vi "Navigation_Main_r1.vi"() -> ()   [LabVIEW 2015]
uses:
  <vilib>/myRIO/Instrument Drivers/Onboard IO/PWM/typedefs/PWM Reference.ctl
  <vilib>/myRIO/Common/Instrument Driver Framework/Utilities/typedefs/myRIO Generic Hardware Reference.ctl
  <vilib>/myRIO/Common/Instrument Driver Framework/Utilities/typedefs/Hardware Version Enum.ctl
  <vilib>/myRIO/Common/Instrument Driver Framework/Utilities/typedefs/myRIO v1.0 Reference.ctl
  <vilib>/myRIO/Common/Instrument Driver Framework/Utilities/typedefs/Generic FPGA Reference.ctl
  <vilib>/myRIO/Common/Instrument Driver Framework/myRIO v1.0/PWM/typedefs/PWM Channels Enum.ctl
  <vilib>/myRIO/Instrument Drivers/Onboard IO/PWM/typedefs/PWM Configuration.ctl
  <vilib>/userdefined/High Color/nirio_resource_hc.ctl
  <vilib>/myRIO/Common/Instrument Driver Framework/myRIO v1.0/PWM/vis/myRIO v1.1 Open PWM.vi
  <vilib>/myRIO/Common/Instrument Driver Framework/Utilities/vis/Validate Channels.vi
  <vilib>/myRIO/Common/Instrument Driver Framework/myRIO v1.0/PWM/vis/myRIO v1.0 Reserve PWM.vi
  <vilib>/myRIO/Common/Instrument Driver Framework/myRIO v1.0/PWM/vis/myRIO v1.0 Close PWM.vi
  <vilib>/myRIO/Common/Instrument Driver Framework/myRIO v1.0/PWM/vis/myRIO v1.0 Build MUX Configuration PWM.vi
  <vilib>/myRIO/Common/Instrument Driver Framework/myRIO v1.0/Resource Manager/vis/myRIO v1.0 Reserve Channel List.vi
  <vilib>/myRIO/Common/Instrument Driver Framework/myRIO v1.0/PWM/vis/myRIO v1.0 Unreserve PWM.vi
  <vilib>/myRIO/Common/Instrument Driver Framework/myRIO v1.0/Resource Manager/vis/myRIO v1.0 Create Configuration List.vi
  <vilib>/myRIO/Common/Instrument Driver Framework/myRIO v1.0/Resource Manager/vis/myRIO v1.0 Reserve Channel.vi
  <vilib>/myRIO/Common/Instrument Driver Framework/myRIO v1.0/Resource Manager/vis/myRIO v1.0 Unreserve Channel.vi
  <vilib>/myRIO/Common/Instrument Driver Framework/myRIO v1.0/Resource Manager/vis/myRIO v1.0 Unreserve Channel List.vi
  <vilib>/myRIO/Common/Instrument Driver Framework/myRIO v1.0/Resource Manager/vis/myRIO v1.0 Build Mutex Name.vi
  <vilib>/FPGAPlugInAG/myRIO-1900/niLvFpga_Open_myRIO-1900.vi
  <vilib>/rvi/interface/common/dynamic/niFpgaDynamicAddResources.vi
  <vilib>/myRIO/Common/Instrument Driver Framework/Utilities/vis/FPGA Ref Manager.vi
  <vilib>/Utility/error.llb/Error Cluster From Error Code.vi
  <vilib>/myRIO/Common/Instrument Driver Framework/Utilities/vis/Ref Counter.vi
  <vilib>/rvi/errors/niLvFpgaAdjustHostInterfaceError.vi
  <vilib>/Utility/VariantDataType/GetNumericInfo.vi
  <vilib>/myRIO/Common/Instrument Driver Framework/myRIO v1.0/myRIO v1.1 Open.vi
  <vilib>/myRIO/Common/Instrument Driver Framework/Utilities/vis/IO Manager.vi
  <vilib>/myRIO/Common/Instrument Driver Framework/Utilities/vis/Configuration Manager.vi
  <vilib>/myRIO/Common/Instrument Driver Framework/myRIO v1.0/Resource Manager/vis/myRIO v1.0 Configure IO.vi
  <vilib>/myRIO/Common/Instrument Driver Framework/myRIO v1.0/myRIO v1.0 Close.vi
  <vilib>/myRIO/Common/Instrument Driver Framework/myRIO v1.0/PWM/vis/myRIO v1.0 Write PWM.vi
  <vilib>/myRIO/Common/Instrument Driver Framework/myRIO v1.0/PWM/vis/myRIO v1.0 Shutdown PWM.vi
  <vilib>/rvi/interface/nirviOpenFPGA/nirviOpenFPGA.xnode
  Navi/E/FPGA Bitfiles/NavigationProjec_FPGATarget2_FPGAMainNavigati_PWPHW8gwDxI.lvbitx
  <vilib>/rvi/interface/nirviReadWriteControl/nirviReadWriteControl.xnode
  <vilib>/myRIO/Instrument Drivers/Onboard IO/PWM/vis/myRIO PWM Open.xnode
  <vilib>/myRIO/Instrument Drivers/Onboard IO/PWM/PWM.lvlib
  <vilib>/myRIO/Instrument Drivers/Utilities/Utilities.lvlib
  NiFpgaLv.dll
  <vilib>/rvi/interface/Simulation/niFpgaSimulationCallBeginRW.vi
panel:
  out "tan(x)":dbl
  in  "x":dbl
  out "X Distance Taveled":dbl
  out "Y Distance Traveled":dbl
  out "Left ENC Avg":dbl
  out "Right ENC Avg":dbl
  out "Distance Traveled":dbl
  out "X Current Position":dbl
  out "Y Current Position":dbl
  out "Reset X Y":dbl
  out "Tick Count(mSec) 2":u32 caption="Tick Count(mSec)"
  out "Right Setpoint":dbl
  out "Left Setpoint":dbl
  out "Scale":dbl=1.0
  in  "Go":bool
  in  "Start Position Y":dbl=5.0
  in  "Goal Position X":dbl=20.0
  in  "Start Position X":dbl=1.0
  in  "All Stop":bool
  in  "Left Side PID Gains":T1={"proportional gain (Kc)"=0.002, "integral time (Ti, min)"=7e-07, "derivative time (Td, min)"=0.0} {"derivative time (Td, min)" format="%.8f"; "integral time (Ti, min)" format="%.8f"; "proportional gain (Kc)" format="%.8f"}
  in  "Left Side Output Range":cluster{"output high":dbl, "output low":dbl}={"output high"=0.13333, "output low"=-0.13333} {"output low" format="%.5f"; "output high" format="%.5f"}
  in  "Right Side PID Gains":T1={"proportional gain (Kc)"=0.002, "integral time (Ti, min)"=7e-07, "derivative time (Td, min)"=0.0} {"derivative time (Td, min)" format="%.8f"; "integral time (Ti, min)" format="%.8f"; "proportional gain (Kc)" format="%.8f"}
  in  "Right Side Output Range":cluster{"output high":dbl, "output low":dbl}={"output high"=0.13333, "output low"=-0.13333} {"output low" format="%.5f"; "output high" format="%.5f"}
  out "Left PWM":dbl
  out "Right PWM":dbl
  out "LF Rot Velocity (rot/s)":dbl
  out "LM Rot Velocity (rot/s)":dbl
  out "LR Rot Velocity (rot/s)":dbl
  out "RR Rot Velocity (rot/s)":dbl
  out "RM Linear Velocity (rot/s)":dbl
  out "RF Linear Velocity (rot/s)":dbl
  in  "Encoder Reset":bool
  out "SYS.SELECTA":u8 format="%08b"
  out "ENC.B_c.CNTR":i32
  out "ENC.B_b.CNTR":i32
  out "ENC.B_a.CNTR":i32
  out "ENC.A_c.CNTR":i32
  out "ENC.A_b.CNTR":i32
  out "ENC.A_a.CNTR":i32
  out "Current Rot Velocity (rot/s)":T2(graph)
  # "Motor Control Parameters"
  # "Press Go when Start and Goal Are Set"
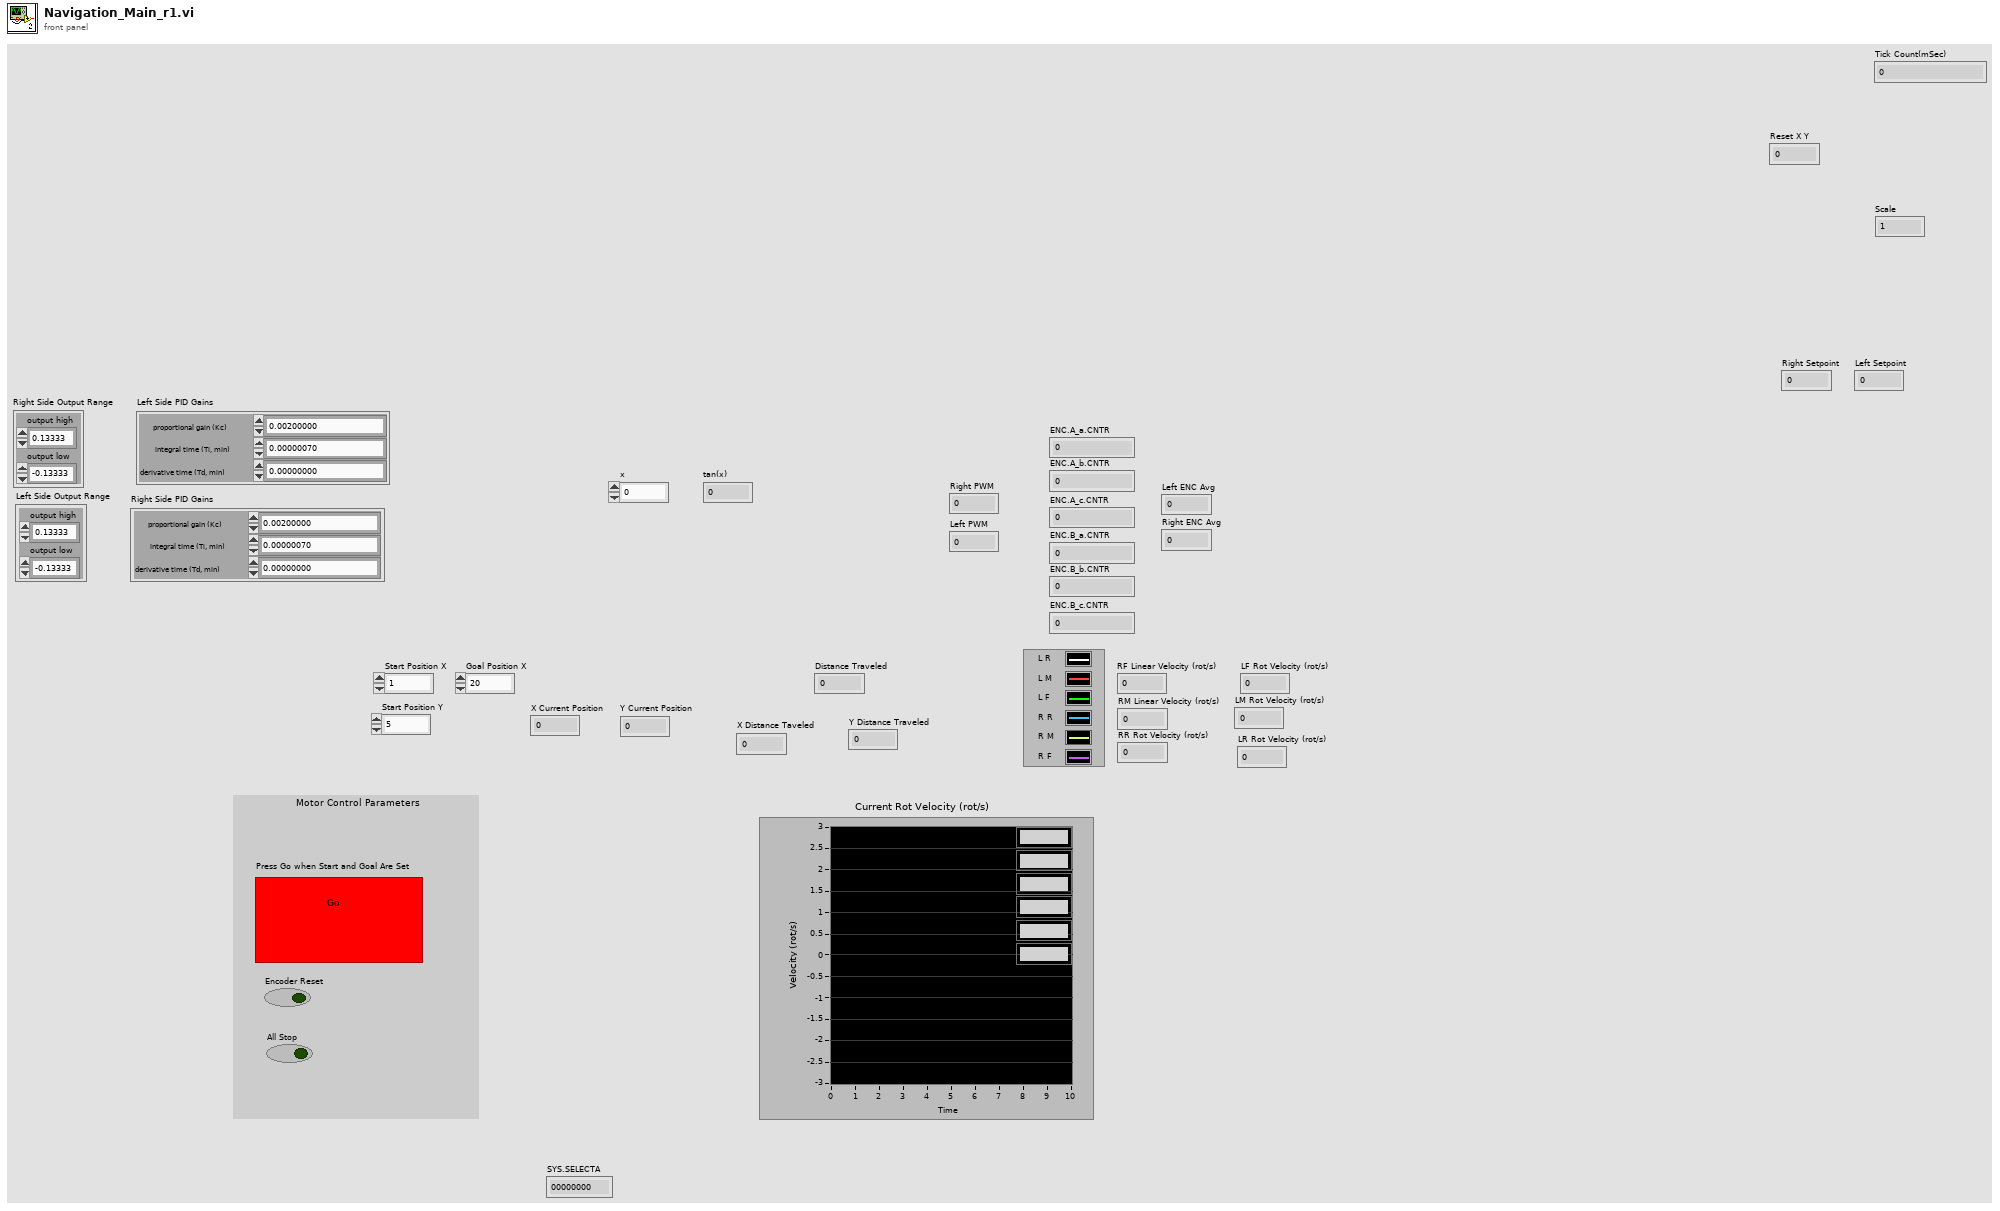
[diagram p1: front panel]
types:
  T1 = cluster{"proportional gain (Kc)":dbl, "integral time (Ti, min)":dbl, "derivative time (Td, min)":dbl}
  T2 = cluster{"Rotational Velocity (RPS)":dbl, "Rotational Velocity (RPS)":dbl, "Rotational Velocity (RPS)":dbl, "Rotational Velocity (RPS)":dbl, "Rotational Velocity (RPS)":dbl, "Rotational Velocity (RPS)":dbl}
  T3 = typedef "nirio_resource_hc.ctl" = tag
  T4 = typedef "Hardware Version Enum.ctl" = enum16{"Unknown", "myRIO-1900", "myRIO-1950", "roboRIO"}
  T5 = typedef "PWM.lvlib/PWM Reference.ctl" = cluster{"myRIO Reference":T6, "PWM Channels Enum":T9, "PWM Configuration":T10}
  T6 = typedef "myRIO Generic Hardware Reference.ctl" = cluster{"myRIO Model":T4, "myRIO Hardware Reference":T7}
  T7 = typedef "myRIO v1.0 Reference.ctl" = cluster{"Generic FPGA Reference":T8, "Allow multiple opens":bool}
  T8 = typedef "Generic FPGA Reference.ctl" = refnum<k20>
  T9 = typedef "PWM Channels Enum.ctl" = enum16{"Not Connected", "C/PWM0", "C/PWM1", "A/PWM0", "A/PWM1", "A/PWM2", "B/PWM0", "B/PWM1", "B/PWM2", "PWM/PWM0", "PWM/PWM1", "PWM/PWM2", "PWM/PWM3", "PWM/PWM4", "PWM/PWM5", "PWM/PWM6", "PWM/PWM7", "PWM/PWM8", "PWM/PWM9"}
  T10 = typedef "PWM.lvlib/PWM Configuration.ctl" = cluster{"Frequency":dbl, "Duty Cycle":dbl}
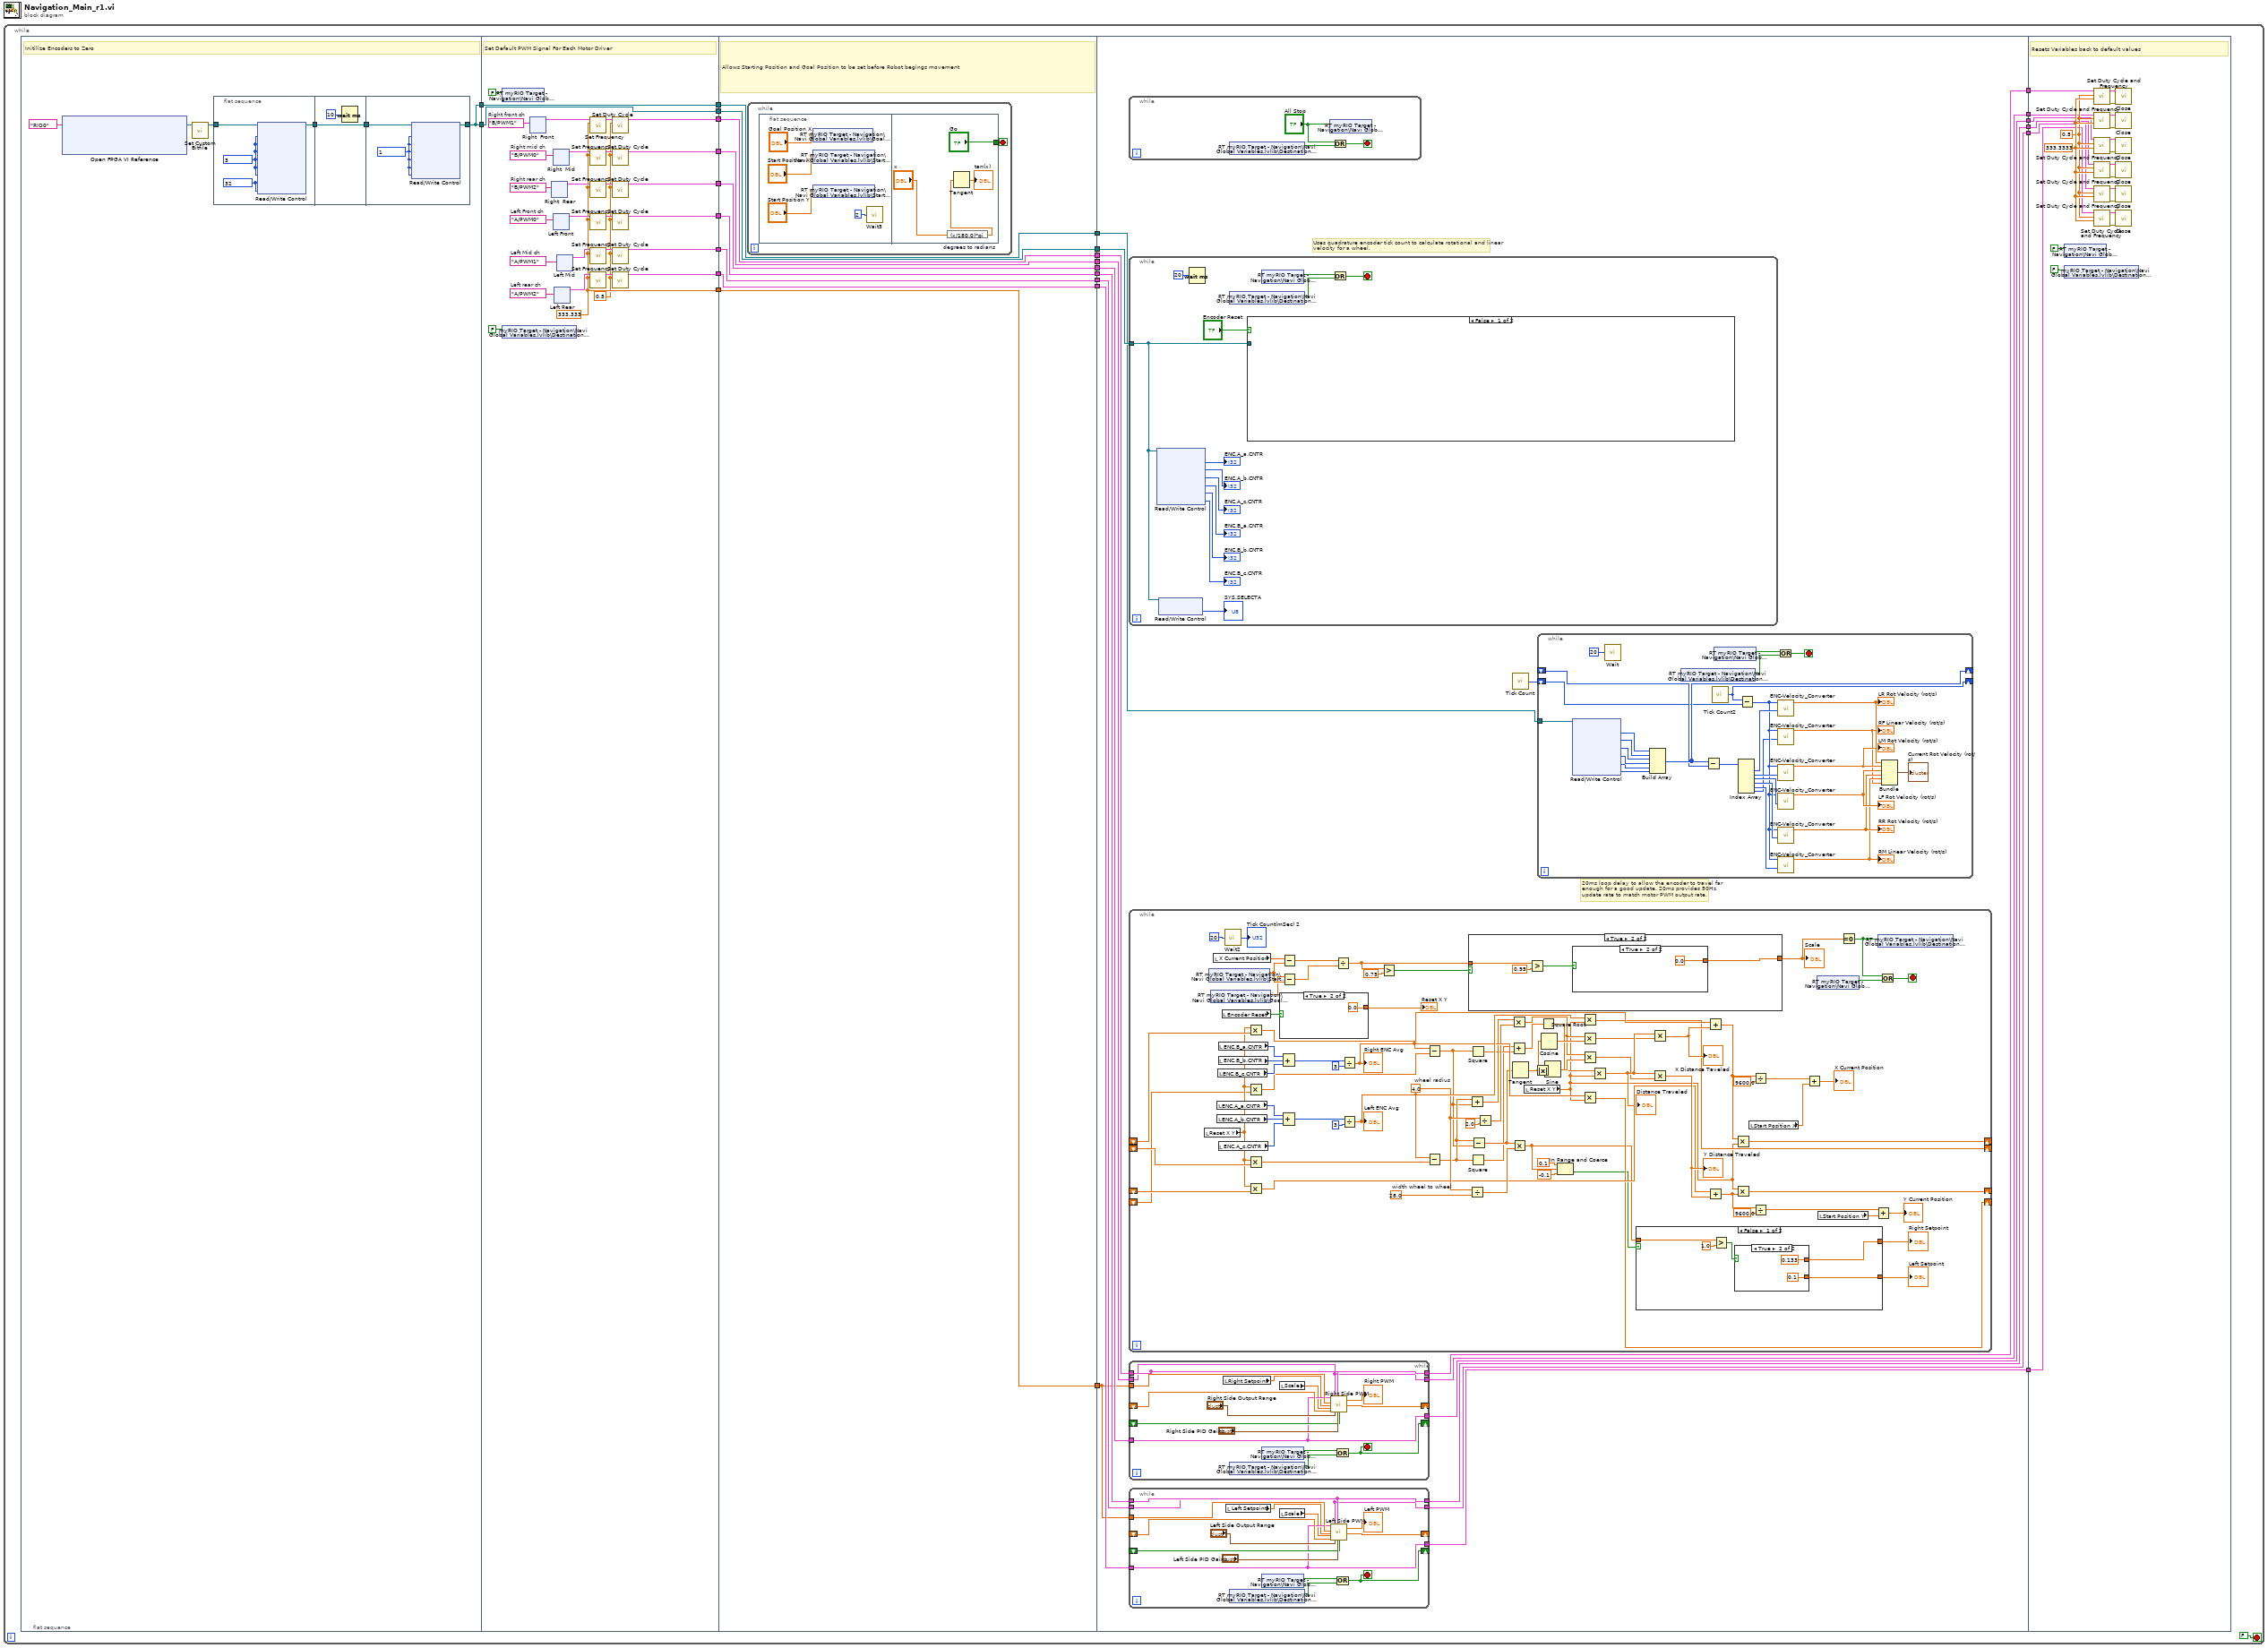
[diagram p0: block diagram]
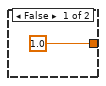
[diagram p2: hidden frame]
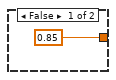
[diagram p3: hidden frame]
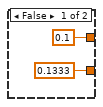
[diagram p4: hidden frame]
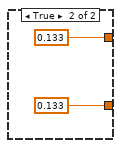
[diagram p5: hidden frame]
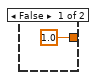
[diagram p6: hidden frame]
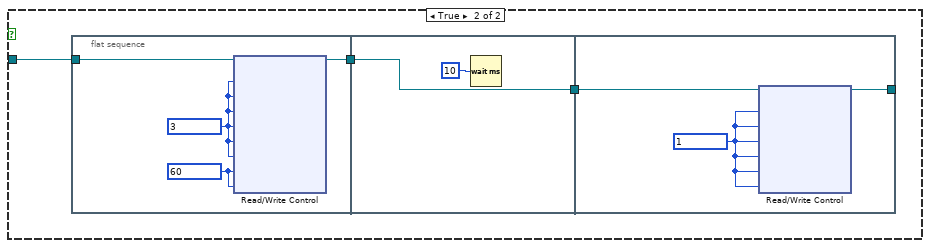
[diagram p7: hidden frame]
diagram:
  n1 = while {
    stop <- FALSE ("stop") stop-if-true
    n2 = flat-sequence {
      tunnel: [w30] -> w27
      tunnel: [w30] -> w26
      tunnel: [w60] -> w25
      tunnel: [w55] -> w24
      tunnel: [w51] -> w23
      tunnel: [w50] -> w22
      tunnel: [w49] -> w21
      tunnel: [w48] -> w20
      tunnel: [w47] -> w19
      tunnel: [w46] -> w18
      tunnel: w27 -> [w45]
      tunnel: [w45] -> w17
      tunnel: w26 -> [w46]
      tunnel: w25 -> [w177]
      tunnel: [w177] -> w16
      tunnel: w24 -> [w176]
      tunnel: [w176] -> w15
      tunnel: w23 -> [w175]
      tunnel: [w175] -> w14
      tunnel: w22 -> [w174]
      tunnel: [w174] -> w13
      tunnel: w21 -> [w173]
      tunnel: [w173] -> w12
      tunnel: w20 -> [w172]
      tunnel: [w172] -> w11
      tunnel: w19 -> [w171]
      tunnel: [w171] -> w10
      tunnel: w18 -> [w170]
      tunnel: [w170] -> w9
      tunnel: w17 -> [w169]
      tunnel: [w169] -> w8
      tunnel: w16 -> [w193]
      tunnel: w15 -> [w194]
      tunnel: w14 -> [w199]
      tunnel: w13 -> [w198]
      tunnel: w12 -> [w197]
      tunnel: w11 -> [w196]
      tunnel: w10 -> [w195]
      tunnel: w9 -> [w201]
      tunnel: w8 -> [w200]
      tunnel: [w192] -> w7
      tunnel: [w191] -> w6
      tunnel: [w190] -> w5
      tunnel: [w189] -> w4
      tunnel: [w188] -> w3
      tunnel: [w187] -> w2
      tunnel: w7 -> [w399]
      tunnel: w6 -> [w398]
      tunnel: w5 -> [w397]
      tunnel: w4 -> [w396]
      tunnel: w3 -> [w395]
      tunnel: w2 -> [w394]
      frame #0 {
        # "Initilize Encoders to Zero"
        n3 = xnode "Open FPGA VI Reference"("resource name"=tag "RIO0") -> ("FPGA VI Reference Out"=w29:refnum<k20>)  [unwired: 1 in, 1 out]
        n4 = call <vilib>:"Set Custom Bitfile.vi"("Custom FPGA Reference In"=w29) -> ("Custom FPGA Reference Out"=w31:refnum<k20>)  [unwired: 9 in, 1 out]
        n5 = flat-sequence {
          tunnel: w31 -> [w36]
          tunnel: [w34] -> w33
          tunnel: w33 -> [w38]
          tunnel: [w38] -> w32
          tunnel: w32 -> [w41]
          tunnel: [w40] -> w30
          frame #0 {
            w35 = u8 32 ("SYS.SELECTA")
            w37 = u8 3 ("ENC.B_c.CNFG")
            n6 = xnode "Read/Write Control"("FPGA VI Reference In"=w36, "ENC.A_a.CNFG"=w37, "ENC.A_b.CNFG"=w37, "ENC.A_c.CNFG"=w37, "ENC.B_a.CNFG"=w37, "ENC.B_b.CNFG"=w37, "ENC.B_c.CNFG"=w37, "SYS.SELECTA"=w35, "SYS.SELECTB"=w35) -> ("FPGA VI Reference Out"=w34:refnum<k20>)  [unwired: 1 in, 1 out]
          }
          frame #1 {
            n7 = Wait (ms)(milliseconds to wait=u32 10) -> ()  [unwired: 1 out]
          }
          frame #2 {
            w42 = u8 1 ("ENC.B_c.CNFG")
            n8 = xnode "Read/Write Control"("FPGA VI Reference In"=w41, "ENC.A_a.CNFG"=w42, "ENC.A_b.CNFG"=w42, "ENC.A_c.CNFG"=w42, "ENC.B_a.CNFG"=w42, "ENC.B_b.CNFG"=w42, "ENC.B_c.CNFG"=w42) -> ("FPGA VI Reference Out"=w40:refnum<k20>)  [unwired: 1 in, 1 out]
          }
        }
      }
      frame #1 {
        w52 = 0.5 ("Duty Cycle")
        w60 = 333.333 ("Frequency [Hz]")
        w67 = tag "B/PWM2"  # Right rear ch
        w68 = tag "B/PWM0"  # Right mid ch
        w69 = tag "B/PWM1"  # Right front ch
        w70 = tag "A/PWM2"  # Left rear ch
        w71 = tag "A/PWM0"  # Left Front ch
        w72 = tag "A/PWM1"  # Left Mid ch
        # "Set Default PWM Signal For Each Motor Driver"
        n9 = shared-variable "RT myRIO Target - Navigation\\Navi Global Variables.lvlib\\All Stop"(FALSE) -> ()  [unwired: 1 in, 1 out]
        n10 = shared-variable "RT myRIO Target - Navigation\\Navi Global Variables.lvlib\\Destination Reached"(FALSE) -> ()  [unwired: 1 in, 1 out]
        n11 = xnode "Right  Front"("Channel Name"=w69) -> ("PWM Ref Out"=w63:T5)  [unwired: 2 in, 1 out]
        n12 = xnode "Right  Rear"("Channel Name"=w67) -> ("PWM Ref Out"=w61:T5)  [unwired: 2 in, 1 out]
        n13 = xnode "Right  Mid"("Channel Name"=w68) -> ("PWM Ref Out"=w62:T5)  [unwired: 2 in, 1 out]
        n14 = xnode "Left Front"("Channel Name"=w71) -> ("PWM Ref Out"=w65:T5)  [unwired: 2 in, 1 out]
        n15 = xnode "Left Rear"("Channel Name"=w70) -> ("PWM Ref Out"=w64:T5)  [unwired: 2 in, 1 out]
        n16 = xnode "Left Mid"("Channel Name"=w72) -> ("PWM Ref Out"=w66:T5)  [unwired: 2 in, 1 out]
        n17 = call <vilib>:"Set Frequency.vi"("Frequency [Hz]"=w60, "PWM Ref In"=w63) -> ("PWM Ref Out"=w56:T5)  [unwired: 7 in, 1 out]
        n18 = call <vilib>:"Set Frequency.vi"("Frequency [Hz]"=w60, "PWM Ref In"=w62) -> ("PWM Ref Out"=w57:T5)  [unwired: 7 in, 1 out]
        n19 = call <vilib>:"Set Frequency.vi"("Frequency [Hz]"=w60, "PWM Ref In"=w61) -> ("PWM Ref Out"=w58:T5)  [unwired: 7 in, 1 out]
        n20 = call <vilib>:"Set Frequency.vi"("Frequency [Hz]"=w60, "PWM Ref In"=w65) -> ("PWM Ref Out"=w53:T5)  [unwired: 7 in, 1 out]
        n21 = call <vilib>:"Set Frequency.vi"("Frequency [Hz]"=w60, "PWM Ref In"=w66) -> ("PWM Ref Out"=w59:T5)  [unwired: 7 in, 1 out]
        n22 = call <vilib>:"Set Frequency.vi"("Frequency [Hz]"=w60, "PWM Ref In"=w64) -> ("PWM Ref Out"=w54:T5)  [unwired: 7 in, 1 out]
        n23 = call <vilib>:"Set Duty Cycle.vi"("Duty Cycle"=w52, "PWM Ref In"=w56) -> ("PWM Ref Out"=w51:T5)  [unwired: 7 in, 1 out]
        n24 = call <vilib>:"Set Duty Cycle.vi"("Duty Cycle"=w52, "PWM Ref In"=w57) -> ("PWM Ref Out"=w50:T5)  [unwired: 7 in, 1 out]
        n25 = call <vilib>:"Set Duty Cycle.vi"("Duty Cycle"=w52, "PWM Ref In"=w58) -> ("PWM Ref Out"=w49:T5)  [unwired: 7 in, 1 out]
        n26 = call <vilib>:"Set Duty Cycle.vi"("Duty Cycle"=w52, "PWM Ref In"=w53) -> ("PWM Ref Out"=w48:T5)  [unwired: 7 in, 1 out]
        n27 = call <vilib>:"Set Duty Cycle.vi"("Duty Cycle"=w52, "PWM Ref In"=w59) -> ("PWM Ref Out"=w47:T5)  [unwired: 7 in, 1 out]
        n28 = call <vilib>:"Set Duty Cycle.vi"("Duty Cycle"=w52, "PWM Ref In"=w54) -> ("PWM Ref Out"=w55:T5)  [unwired: 7 in, 1 out]
      }
      frame #2 {
        # "Allows Starting Position and Goal Position to be set before Robot begings movement"
        n29 = while {
          stop <- w178 stop-if-true
          n30 = flat-sequence {
            tunnel: ["Go"] -> w178
            frame #0 {
              n31 = shared-variable "RT myRIO Target - Navigation\\Navi Global Variables.lvlib\\Goal Position X"("Goal Position X") -> ()  [unwired: 1 in, 1 out]
              n32 = shared-variable "RT myRIO Target - Navigation\\Navi Global Variables.lvlib\\Start Position X"("Start Position X") -> ()  [unwired: 1 in, 1 out]
              n33 = shared-variable "RT myRIO Target - Navigation\\Navi Global Variables.lvlib\\Start Position Y"("Start Position Y") -> ()  [unwired: 1 in, 1 out]
              n34 = call "Wait3"("Count(mSec)"=u32 2) -> ()  [unwired: 1 out]
            }
            frame #1 {
              n35 = expression code="(x/180.0)*pi" "degrees to radians"("x") -> (w183:dbl)
              n36 = Tangent(1:w183) -> (0:→"tan(x)":dbl)
            }
          }
        }
      }
      frame #3 {
        # "Uses quadrature encoder tick count to calculate rotational and linear velocity for a wheel."
        # "20ms loop delay to allow the encoder to travel far enough for a good update. 20ms provides 50Hz update rate to match motor PWM output rate."
        n37 = while {
          stop <- w306 stop-if-true
          n38 = shared-variable "RT myRIO Target - Navigation\\Navi Global Variables.lvlib\\Destination Reached"() -> (w304:bool)  [unwired: 1 in, 1 out]
          n39 = shared-variable "RT myRIO Target - Navigation\\Navi Global Variables.lvlib\\All Stop"("All Stop") -> ()  [unwired: 1 in, 1 out]
          n40 = Or(x="All Stop", y=w304) -> (x .or. y?=w306:bool)
        }
        n41 = while {
          tunnel: w201 -> [w340]
          stop <- w337 stop-if-true
          n42 = xnode "Read/Write Control"("FPGA VI Reference In"=w340) -> ("ENC.A_a.CNTR"=→"ENC.A_a.CNTR":u32, "ENC.A_b.CNTR"=→"ENC.A_b.CNTR":u32, "ENC.A_c.CNTR"=→"ENC.A_c.CNTR":u32, "ENC.B_a.CNTR"=→"ENC.B_a.CNTR":u32, "ENC.B_b.CNTR"=→"ENC.B_b.CNTR":u32, "ENC.B_c.CNTR"=→"ENC.B_c.CNTR":u32)  [unwired: 1 in, 2 out]
          n43 = xnode "Read/Write Control"("FPGA VI Reference In"=w340) -> ("SYS.SELECTA"=→"SYS.SELECTA":u8)  [unwired: 1 in, 2 out]
          n44 = Wait (ms)(milliseconds to wait=u32 20) -> ()  [unwired: 1 out]
          n45 = shared-variable "RT myRIO Target - Navigation\\Navi Global Variables.lvlib\\Destination Reached"() -> (w339:bool)  [unwired: 1 in, 1 out]
          n46 = case shown="False" "Encoder Reset" {
            tunnel: w340 -> [_ w350]
            frame False {
            }
            frame True {
              n47 = flat-sequence {
                tunnel: w350 -> [w355]
                tunnel: [w353] -> w352
                tunnel: w352 -> [w357]
                tunnel: [w357] -> w351
                tunnel: w351 -> [w360]
                tunnel: [w359] -> _
                frame #0 {
                  w354 = u8 60 ("SYS.SELECTA")
                  w356 = u8 3 ("ENC.B_c.CNFG")
                  n48 = xnode "Read/Write Control"("FPGA VI Reference In"=w355, "ENC.A_a.CNFG"=w356, "ENC.A_b.CNFG"=w356, "ENC.A_c.CNFG"=w356, "ENC.B_a.CNFG"=w356, "ENC.B_b.CNFG"=w356, "ENC.B_c.CNFG"=w356, "SYS.SELECTA"=w354, "SYS.SELECTB"=w354) -> ("FPGA VI Reference Out"=w353:refnum<k20>)  [unwired: 1 in, 1 out]
                }
                frame #1 {
                  n49 = Wait (ms)(milliseconds to wait=u32 10) -> ()  [unwired: 1 out]
                }
                frame #2 {
                  w361 = u8 1 ("ENC.B_c.CNFG")
                  n50 = xnode "Read/Write Control"("FPGA VI Reference In"=w360, "ENC.A_a.CNFG"=w361, "ENC.A_b.CNFG"=w361, "ENC.A_c.CNFG"=w361, "ENC.B_a.CNFG"=w361, "ENC.B_b.CNFG"=w361, "ENC.B_c.CNFG"=w361) -> ("FPGA VI Reference Out"=w359:refnum<k20>)  [unwired: 1 in, 1 out]
                }
              }
            }
          }
          n51 = shared-variable "RT myRIO Target - Navigation\\Navi Global Variables.lvlib\\All Stop"() -> (w338:bool)  [unwired: 1 in, 1 out]
          n52 = Or(x=w338, y=w339) -> (x .or. y?=w337:bool)
        }
        n53 = while {
          shift-right: [w237] -> _
          shift-left: _ -> [w271]
          shift-right: [w234] -> _
          shift-left: _ -> [w204]
          shift-right: [w236] -> _
          shift-left: _ -> [w249]
          shift-right: [w235] -> _
          shift-left: _ -> [w248]
          stop <- w214 stop-if-true
          w267 = 28.0  # width wheel to wheel
          w268 = 4.0  # wheel radius
          n54 = local read "Reset X Y"() -> (w233:dbl)
          n55 = shared-variable "RT myRIO Target - Navigation\\Navi Global Variables.lvlib\\Start Position X"() -> (w211:dbl)  [unwired: 1 in, 1 out]
          n56 = shared-variable "RT myRIO Target - Navigation\\Navi Global Variables.lvlib\\Goal Position X"() -> (w210:dbl)  [unwired: 1 in, 1 out]
          n57 = local read "X Current Position"() -> (w222:dbl)
          n58 = local read "ENC.A_a.CNTR"() -> (w279:i32)
          n59 = local read "ENC.A_b.CNTR"() -> (w278:i32)
          n60 = local read "ENC.B_c.CNTR"() -> (w274:i32)
          n61 = local read "ENC.B_a.CNTR"() -> (w276:i32)
          n62 = local read "ENC.B_b.CNTR"() -> (w275:i32)
          n63 = local read "ENC.A_c.CNTR"() -> (w277:i32)
          n64 = local read "Encoder Reset"() -> (w230:bool)
          n65 = call "Wait2"("Count(mSec)"=u32 20) -> ("Tick Count(mSec)"=→"Tick Count(mSec) 2":u32)
          n66 = Multiply(x=w233, y=w248) -> (x*y=w239:dbl)
          n67 = Multiply(x=w233, y=w204) -> (x*y=w238:dbl)
          n68 = Multiply(x=w233, y=w271) -> (x*y=w241:dbl)
          n69 = Multiply(x=w233, y=w249) -> (x*y=w240:dbl)
          n70 = case shown="True" w230 {
            tunnel: [1.0 0.0] -> w212
            frame False {
            }
            frame True {
            }
          }
          "Reset X Y" <- w212
          n71 = Subtract(x=w222, y=w211) -> (x-y=w218:dbl)
          n72 = Subtract(x=w210, y=w211) -> (x-y=w217:dbl)
          n73 = Compound Arithmetic op=ADD(w276, w275, w274) -> (w282:i32)
          n74 = Compound Arithmetic op=ADD(w279, w278, w277) -> (w283:i32)
          n75 = Divide(x=w218, y=w217) -> (x/y=w219:dbl)
          n76 = Divide(x=w282, y=3) -> (x/y=w270:dbl)
          "Right ENC Avg" <- w270
          n77 = Divide(x=w283, y=3) -> (x/y=w272:dbl)
          "Left ENC Avg" <- w272
          n78 = Greater?(x=w219, y=0.75) -> (0:w220:bool)
          n79 = Subtract(x=w270, y=w238) -> (x-y=w261:dbl)
          n80 = Subtract(x=w272, y=w241) -> (x-y=w262:dbl)
          n81 = case shown="True" w220 {
            tunnel: w219 -> [_ w288]
            tunnel: [1.0 w285] -> w213
            frame False {
            }
            frame True {
              n82 = Greater?(x=w288, y=0.95) -> (0:w286:bool)
              n83 = case shown="True" w286 {
                tunnel: [0.85 0.0] -> w285
                frame False {
                }
                frame True {
                }
              }
            }
          }
          "Scale" <- w213
          n84 = Add(x=w262, y=w261) -> (x+y=w265:dbl)
          n85 = Divide(x=w268, y=w267) -> (x/y=w263:dbl)
          n86 = Square(x=w261) -> (x^2=w260:dbl)
          n87 = Square(x=w262) -> (x^2=w259:dbl)
          n88 = Subtract(x=w262, y=w261) -> (x-y=w264:dbl)
          n89 = Divide(x=w268, y=2.0) -> (x/y=w266:dbl)
          n90 = Multiply(x=w265, y=w266) -> (x*y=w255:dbl)
          n91 = Add(x=w259, y=w260) -> (x+y=w258:dbl)
          n92 = Multiply(x=w264, y=w263) -> (x*y=w223:dbl)
          n93 = Tangent(1:w264) -> (0:w207:dbl)
          n94 = local read "Reset X Y"() -> (w231:dbl)
          n95 = Absolute Value(x=w207) -> (abs(x)=w203:dbl)
          n96 = Square Root(x=w258) -> (sqrt(x)=w254:dbl)
          n97 = Cosine(x=w207) -> (cos(x)=w256:dbl)
          n98 = Sine(x=w203) -> (sin(x)=w257:dbl)
          n99 = In Range and Coerce(upper limit=0.1, x=w223, lower limit=-0.1) -> (In Range?=w224:bool)  [unwired: 1 out]
          n100 = Multiply(x=w272, y=w231) -> (x*y=w237:dbl)
          n101 = Multiply(x=w255, y=w256) -> (x*y=w206:dbl)
          n102 = Multiply(x=w255, y=w257) -> (x*y=w205:dbl)
          n103 = Multiply(x=w270, y=w231) -> (x*y=w234:dbl)
          n104 = Multiply(x=w254, y=w231) -> (x*y=w232:dbl)
          "Distance Traveled" <- w232
          n105 = case shown="False" w224 {
            tunnel: w223 -> [w295 _]
            tunnel: [w292 0.133] -> w209
            tunnel: [w291 0.133] -> w208
            frame False {
              n106 = Greater?(x=w295, y=1.0) -> (0:w293:bool)
              n107 = case shown="True" w293 {
                tunnel: [0.1333 0.1] -> w292
                tunnel: [0.1 0.133] -> w291
                frame False {
                }
                frame True {
                }
              }
            }
            frame True {
            }
          }
          "Left Setpoint" <- w209
          "Right Setpoint" <- w208
          n108 = Multiply(x=w232, y=w206) -> (x*y=w253:dbl)
          "X Distance Taveled" <- w253
          n109 = Multiply(x=w232, y=w205) -> (x*y=w252:dbl)
          "Y Distance Traveled" <- w252
          n110 = Add(x=w239, y=w253) -> (x+y=w251:dbl)
          n111 = Add(x=w240, y=w252) -> (x+y=w243:dbl)
          n112 = Multiply(x=w251, y=w231) -> (x*y=w235:dbl)
          n113 = Multiply(x=w231, y=w243) -> (x*y=w236:dbl)
          n114 = local read "Start Position X"() -> (w244:dbl)
          n115 = Divide(x=w251, y=9600.0) -> (x/y=w246:dbl)
          n116 = Divide(x=w243, y=9600.0) -> (x/y=w247:dbl)
          n117 = Add(x=w246, y=w244) -> (x+y=→"X Current Position":dbl)
          n118 = shared-variable "RT myRIO Target - Navigation\\Navi Global Variables.lvlib\\All Stop"() -> (w216:bool)  [unwired: 1 in, 1 out]
          n119 = local read "Start Position Y"() -> (w245:dbl)
          n120 = Equal To 0?(x=w213) -> (x = 0?=w215:bool)
          n121 = Add(x=w247, y=w245) -> (x+y=→"Y Current Position":dbl)
          n122 = shared-variable "RT myRIO Target - Navigation\\Navi Global Variables.lvlib\\Destination Reached"(w215) -> ()  [unwired: 1 in, 1 out]
          n123 = Or(x=w215, y=w216) -> (x .or. y?=w214:bool)
        }
        n124 = while {
          tunnel: w199 -> [w329]
          tunnel: w198 -> [w328]
          tunnel: w197 -> [w327]
          tunnel: w193 -> [w336]
          shift-right: [w332] -> _
          shift-left: _ -> [w331]
          shift-right: [w324] -> _
          shift-left: _ -> [w330]
          tunnel: [w329] -> w192
          tunnel: [w328] -> w191
          tunnel: [w327] -> w190
          stop <- w324 stop-if-true
          n125 = local read "Right Setpoint"() -> (w323:dbl)
          n126 = shared-variable "RT myRIO Target - Navigation\\Navi Global Variables.lvlib\\Destination Reached"() -> (w326:bool)  [unwired: 1 in, 1 out]
          n127 = shared-variable "RT myRIO Target - Navigation\\Navi Global Variables.lvlib\\All Stop"() -> (w325:bool)  [unwired: 1 in, 1 out]
          n128 = local read "Scale"() -> (w322:dbl)
          n129 = call "Right Side PWM.vi"("Right rear"=w327, "Frequency"=w336, "Right Side Setpoint"=w323, "Right Side Scale"=w322, "Right PID Feedback"=w331, "Right Mid"=w328, "Right Side Output Range"="Right Side Output Range", "Right Front"=w329, "Right Side PID Gains"="Right Side PID Gains", "Reset Right E.T."=w330) -> ("Right PWM"=→"Right PWM":dbl, "Right PID Output"=w332:dbl)  [unwired: 8 in]
          n130 = Or(x=w325, y=w326) -> (x .or. y?=w324:bool)
        }
        n131 = while {
          tunnel: w196 -> [w314]
          tunnel: w195 -> [w313]
          tunnel: w194 -> [w312]
          tunnel: w193 -> [w321]
          shift-right: [w317] -> _
          shift-left: _ -> [w316]
          shift-right: [w309] -> _
          shift-left: _ -> [w315]
          tunnel: [w314] -> w189
          tunnel: [w313] -> w188
          tunnel: [w312] -> w187
          stop <- w309 stop-if-true
          n132 = local read "Left Setpoint"() -> (w307:dbl)
          n133 = shared-variable "RT myRIO Target - Navigation\\Navi Global Variables.lvlib\\Destination Reached"() -> (w311:bool)  [unwired: 1 in, 1 out]
          n134 = shared-variable "RT myRIO Target - Navigation\\Navi Global Variables.lvlib\\All Stop"() -> (w310:bool)  [unwired: 1 in, 1 out]
          n135 = local read "Scale"() -> (w308:dbl)
          n136 = call "Left Side PWM.vi"("Left rear"=w312, "Frequency"=w321, "Left Side Setpoint"=w307, "Left Side Scale"=w308, "Left PID Feedback"=w316, "Left Mid"=w313, "Left Side Output Range"="Left Side Output Range", "Left Front"=w314, "Left Side PID Gains"="Left Side PID Gains", "Reset Left E.T."=w315) -> ("Left PWM"=→"Left PWM":dbl, "Left PID Output"=w317:dbl)  [unwired: 8 in]
          n137 = Or(x=w310, y=w311) -> (x .or. y?=w309:bool)
        }
        n138 = call "Tick Count"() -> ("Tick Count(uSec)"=w202:u32)
        n139 = while {
          shift-right: [w383] -> _
          shift-left: _ -> [w382]
          shift-right: [w380] -> _
          shift-left: w202 -> [w379]
          tunnel: w200 -> [w390]
          stop <- w375 stop-if-true
          n140 = xnode "Read/Write Control"("FPGA VI Reference In"=w390) -> ("ENC.A_a.CNTR"=w389:u32, "ENC.A_b.CNTR"=w388:u32, "ENC.A_c.CNTR"=w387:u32, "ENC.B_a.CNTR"=w386:u32, "ENC.B_b.CNTR"=w385:u32, "ENC.B_c.CNTR"=w384:u32)  [unwired: 1 in, 2 out]
          n141 = call "Wait"("Count(mSec)"=u32 20) -> ()  [unwired: 1 out]
          n142 = Build Array(w389, w388, w387, w386, w385, w384) -> (w383:u32[])
          n143 = shared-variable "RT myRIO Target - Navigation\\Navi Global Variables.lvlib\\Destination Reached"() -> (w377:bool)  [unwired: 1 in, 1 out]
          n144 = Subtract(x=w383, y=w382) -> (x-y=w381:u32[])
          n145 = call "Tick Count2"() -> ("Tick Count(uSec)"=w380:u32)
          n146 = shared-variable "RT myRIO Target - Navigation\\Navi Global Variables.lvlib\\All Stop"() -> (w376:bool)  [unwired: 1 in, 1 out]
          n147 = Index Array(array=w381) -> (element #1=w374:u32, element #2=w371:u32, element #3=w369:u32, element #4=w367:u32, element #5=w365:u32, element #6=w362:u32)  [unwired: 6 in]
          n148 = Subtract(x=w380, y=w379) -> (x-y=w363:u32)
          n149 = Or(x=w376, y=w377) -> (x .or. y?=w375:bool)
          n150 = call "ENC-Velocity_Converter.vi"("delta  Encoder Count"=w374, "dt (uSec)"=w363) -> ("Rotational Velocity (RPS)"=w373:dbl)  [unwired: 7 in, 2 out]
          "LR Rot Velocity (rot/s)" <- w373
          n151 = call "ENC-Velocity_Converter.vi"("delta  Encoder Count"=w362, "dt (uSec)"=w363) -> ("Rotational Velocity (RPS)"=w364:dbl)  [unwired: 7 in, 2 out]
          "RF Linear Velocity (rot/s)" <- w364
          n152 = call "ENC-Velocity_Converter.vi"("delta  Encoder Count"=w371, "dt (uSec)"=w363) -> ("Rotational Velocity (RPS)"=w372:dbl)  [unwired: 7 in, 2 out]
          "LM Rot Velocity (rot/s)" <- w372
          n153 = call "ENC-Velocity_Converter.vi"("delta  Encoder Count"=w369, "dt (uSec)"=w363) -> ("Rotational Velocity (RPS)"=w370:dbl)  [unwired: 7 in, 2 out]
          "LF Rot Velocity (rot/s)" <- w370
          n154 = call "ENC-Velocity_Converter.vi"("delta  Encoder Count"=w367, "dt (uSec)"=w363) -> ("Rotational Velocity (RPS)"=w368:dbl)  [unwired: 7 in, 2 out]
          "RR Rot Velocity (rot/s)" <- w368
          n155 = call "ENC-Velocity_Converter.vi"("delta  Encoder Count"=w365, "dt (uSec)"=w363) -> ("Rotational Velocity (RPS)"=w366:dbl)  [unwired: 7 in, 2 out]
          "RM Linear Velocity (rot/s)" <- w366
          n156 = Bundle("Rotational Velocity (RPS)"=w373, "Rotational Velocity (RPS)"=w372, "Rotational Velocity (RPS)"=w370, "Rotational Velocity (RPS)"=w368, "Rotational Velocity (RPS)"=w366, "Rotational Velocity (RPS)"=w364) -> (→"Current Rot Velocity (rot/s)":T2)  [unwired: 1 in]
        }
      }
      frame #4 {
        w400 = 0.5
        w401 = 333.3333
        # "Resets Variables back to default values"
        n157 = shared-variable "RT myRIO Target - Navigation\\Navi Global Variables.lvlib\\All Stop"(FALSE) -> ()  [unwired: 1 in, 1 out]
        n158 = shared-variable "RT myRIO Target - Navigation\\Navi Global Variables.lvlib\\Destination Reached"(FALSE) -> ()  [unwired: 1 in, 1 out]
        n159 = call <vilib>:"Set Duty Cycle and Frequency.vi"("Frequency [Hz]"=w401, "Duty Cycle"=w400, "PWM Ref In"=w399) -> ("error out"=w406:errorcluster, "PWM Ref Out"=w413:T5)  [unwired: 6 in]
        n160 = call <vilib>:"Set Duty Cycle and Frequency.vi"("Frequency [Hz]"=w401, "Duty Cycle"=w400, "PWM Ref In"=w398) -> ("error out"=w411:errorcluster, "PWM Ref Out"=w412:T5)  [unwired: 6 in]
        n161 = call <vilib>:"Set Duty Cycle and Frequency.vi"("Frequency [Hz]"=w401, "Duty Cycle"=w400, "PWM Ref In"=w397) -> ("error out"=w405:errorcluster, "PWM Ref Out"=w410:T5)  [unwired: 6 in]
        n162 = call <vilib>:"Set Duty Cycle and Frequency.vi"("Frequency [Hz]"=w401, "Duty Cycle"=w400, "PWM Ref In"=w396) -> ("error out"=w404:errorcluster, "PWM Ref Out"=w409:T5)  [unwired: 6 in]
        n163 = call <vilib>:"Set Duty Cycle and Frequency.vi"("Frequency [Hz]"=w401, "Duty Cycle"=w400, "PWM Ref In"=w395) -> ("error out"=w403:errorcluster, "PWM Ref Out"=w408:T5)  [unwired: 6 in]
        n164 = call <vilib>:"Set Duty Cycle and Frequency.vi"("Frequency [Hz]"=w401, "Duty Cycle"=w400, "PWM Ref In"=w394) -> ("error out"=w402:errorcluster, "PWM Ref Out"=w407:T5)  [unwired: 6 in]
        n165 = call <vilib>:"Close.vi"("error in (no error)"=w406, "PWM Ref In"=w413) -> ()  [unwired: 9 in, 1 out]
        n166 = call <vilib>:"Close.vi"("error in (no error)"=w411, "PWM Ref In"=w412) -> ()  [unwired: 9 in, 1 out]
        n167 = call <vilib>:"Close.vi"("error in (no error)"=w405, "PWM Ref In"=w410) -> ()  [unwired: 9 in, 1 out]
        n168 = call <vilib>:"Close.vi"("error in (no error)"=w404, "PWM Ref In"=w409) -> ()  [unwired: 9 in, 1 out]
        n169 = call <vilib>:"Close.vi"("error in (no error)"=w403, "PWM Ref In"=w408) -> ()  [unwired: 9 in, 1 out]
        n170 = call <vilib>:"Close.vi"("error in (no error)"=w402, "PWM Ref In"=w407) -> ()  [unwired: 9 in, 1 out]
      }
    }
  }
